vi "Receive Response.vi"(8 "error in (no error)":errorcluster, 10 "Command in":T1, 11 "Laser in":refnum<class "Laser.lvclass">) -> (0 "error out":errorcluster, 2 "Response":string, 3 "Laser out":refnum<class "Laser.lvclass">)   [LabVIEW 2018, in "Laser.lvlib" / "Laser.lvclass"]
doc: "Read response data from laser"
uses:
  Laser.lvclass
  Custom Controls/Command List.ctl
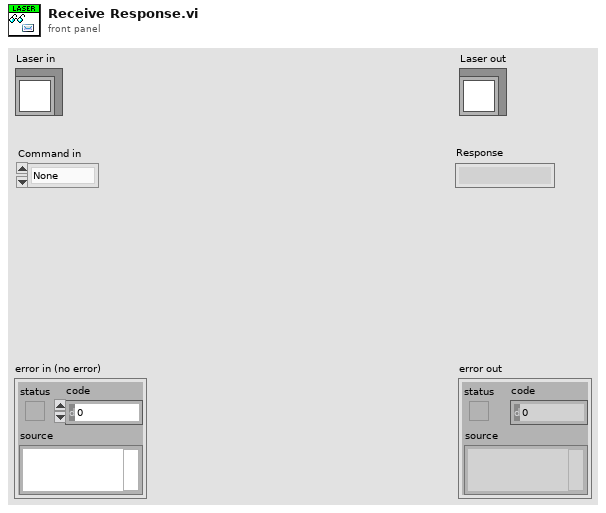
[diagram p1: front panel]
types:
  T1 = typedef "Laser.lvlib/Laser.lvclass/Command List.ctl" = enum16{"None", "Config?", "Volt?", "ThCase?", "STS?", "Mon?", "Help?", "HB", "Verbose", "Spnt", "Ext", "PRF", "Start", "Stop", "PRF?", "State?", "Status?", "Stat?", "Read HB", "Logon", "Poutmax", "saveconfig", "Reset", "Poutmax?", "PoutCommandMax", "PoutCommandMax?", "FreqMin", "FreqMin?"}
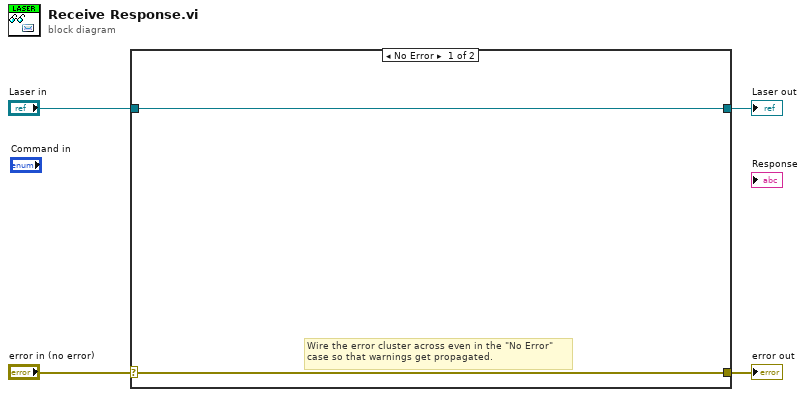
[diagram p0: block diagram]
diagram:
  n1 = case shown="No Error" "error in (no error)" {
    selector: "error in (no error)" -> [w5 w8]
    tunnel: [w5 w8] -> w3
    tunnel: [w6 w7] -> w1
    tunnel: "Laser in" -> [w6 w7]
    frame No Error {
      # "Wire the error cluster across even in the \"No Error\"\ncase so that warnings get propagated."
    }
    frame Error {
    }
  }
  "error out" <- w3
  "Laser out" <- w1
